vi "sub_load_puzzles.vi"(8 "error in (no error)":errorcluster) -> (0 "error out":errorcluster, 3 "puzzles (out)":string[][](array[string]))   [LabVIEW 2018]
uses:
  <vilib>/Utility/file.llb/Read Delimited Spreadsheet (string).vi
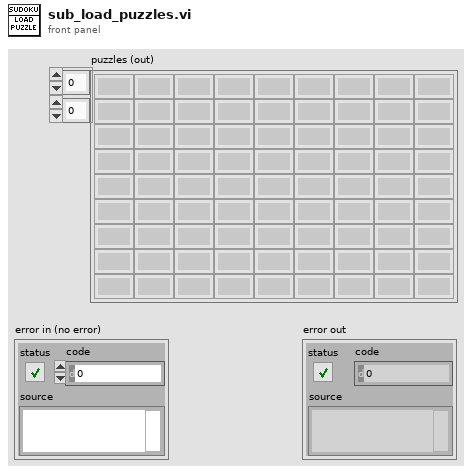
[diagram p1: front panel]
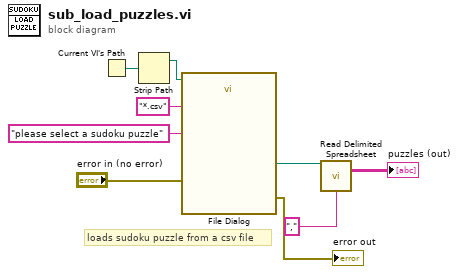
[diagram p0: block diagram]
diagram:
  # "loads sudoku puzzle from a csv file"
  n1 = Current VI's Path() -> (path=w9:path)
  n2 = Strip Path(path=w9) -> (stripped path=w8:path)  [unwired: 1 out]
  n3 = call "File Dialog"("start path"=w8, "prompt"="please select a sudoku puzzle", "error in"="error in (no error)", "pattern (all files)"="*.csv" ("pattern")) -> ("selected path"=w4:path, "error out"=→"error out":errorcluster)  [unwired: 8 in, 2 out]
  n4 = call-poly <vilib>:"Read Delimited Spreadsheet.vi"("file path (dialog if empty)"=w4, "delimiter (\\t)"="," ("delimiter (\\t)")) -> ("all rows"=→"puzzles (out)":string[][])  [unwired: 8 in, 5 out]
